vi "Keithley 2420 read resistance.vi"() -> ()   [LabVIEW 2014]
uses:
  Environmental Chamber LabVIEW and Instruments/Drivers and Software/LabVIEW 8.2 Drivers/keithley_24xx/Keithley 24XX/Public/Data/Read (Single Point).vi
  <vilib>/Utility/file.llb/Write To Spreadsheet File (string).vi
  Environmental Chamber LabVIEW and Instruments/Drivers and Software/keithley_24xx/Keithley 24XX/Keithley 24XX.lvlib
panel:
  in  "save?":bool
  in  "note":string
  in  "Stop Button":bool
  out "K-2420 2":cluster{"Resistance":sgl}(graph)
  in  "K2420 Applied Voltage (V)":dbl=0.1
  in  "K2420-range":dbl=1.0 format="%#_13g"
  in  "Enable Auto Range (T:Enable)":bool=TRUE
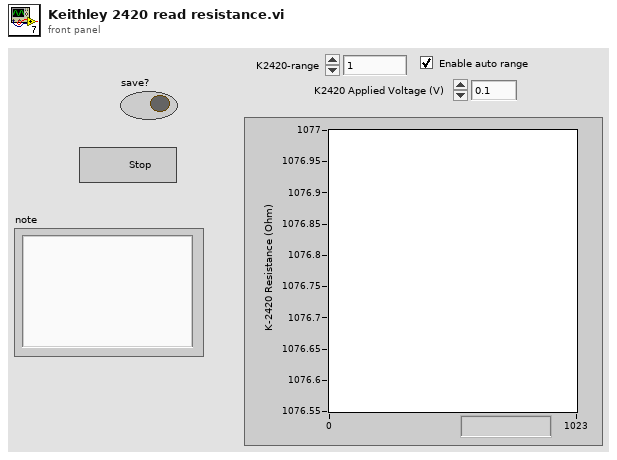
[diagram p1: front panel]
types:
  T1 = enum16{"open", "open or create", "create or replace", "create", "open (read only)"}
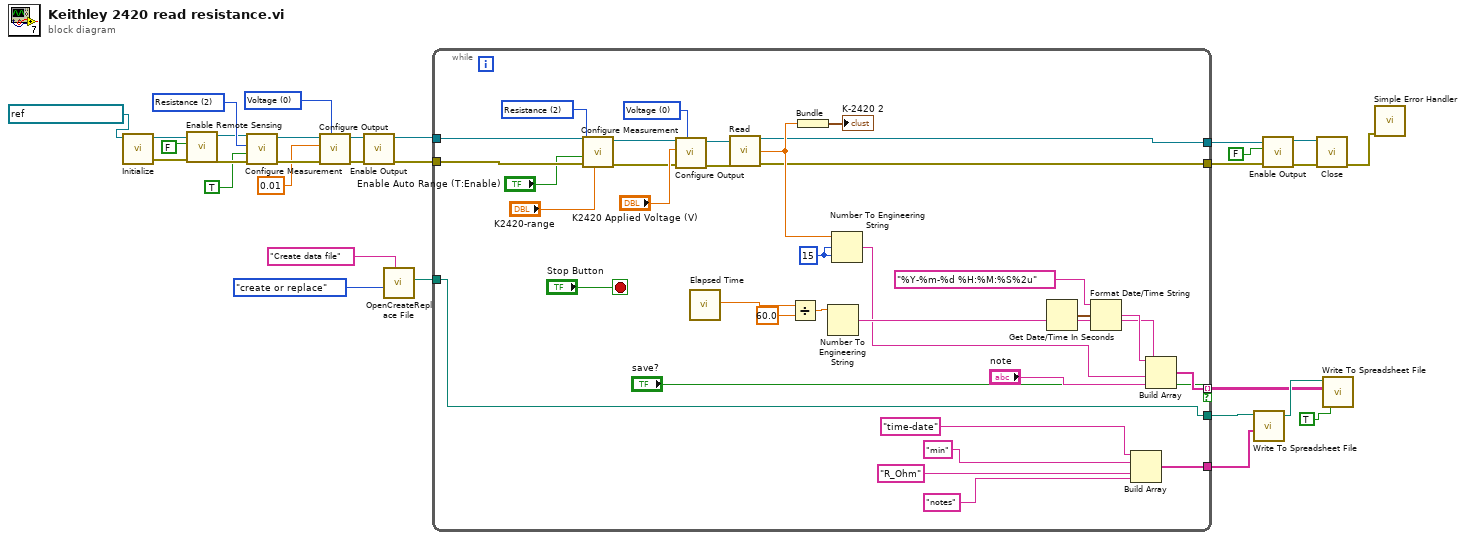
[diagram p0: block diagram]
diagram:
  w15 = u16 0 items=["Voltage", "Current"] ("Source Mode  (0: Voltage)")
  w20 = u16 2 items=["Volts", "Current", "Resistance"] ("Function (0: Volts)")
  n1 = call "Initialize.vi"("VISA resource name"=refnum<visa-resource-name> "GPIB1::24::INSTR") -> ("error out"=w11:errorcluster, "VISA resource name out"=w14:refnum<visa-resource-name>)  [unwired: 9 in]
  n2 = call "Enable Remote Sensing.vi"("error in (no error)"=w11, "Enable Remote Sensing (T: Enable)"=FALSE ("4-wire?"), "VISA resource name"=w14) -> ("error out"=w12:errorcluster, "VISA resource name out"=w13:refnum<visa-resource-name>)  [unwired: 7 in]
  n3 = call "Configure Measurement.vi"("error in (no error)"=w12, "Enable Auto Range (T:Enable)"=TRUE, "Function (0: Volts)"=w20, "VISA resource name"=w13) -> ("error out"=w19:errorcluster, "VISA resource name out"=w18:refnum<visa-resource-name>)  [unwired: 6 in]
  n4 = call "Configure Output.vi"("Source Mode  (0: Voltage)"=w15, "error in (no error)"=w19, "Output Level (0)"=0.01 ("K2420 Applied Voltage (V) 2"), "VISA resource name"=w18) -> ("error out"=w17:errorcluster, "VISA resource name out"=w16:refnum<visa-resource-name>)  [unwired: 6 in]
  n5 = call "Enable Output.vi"("error in (no error)"=w17, "VISA resource name"=w16) -> ("error out"=w29:errorcluster, "VISA resource name out"=w30:refnum<visa-resource-name>)  [unwired: 8 in]
  n6 = call "OpenCreateReplace File.vi"("prompt"="Create data file", "function (open:0)"=T1."create or replace") -> ("new file path"=w22:path)  [unwired: 6 in, 3 out]
  n7 = while {
    tunnel: [w62] -> w24 mode=indexing if="save?"
    tunnel: w30 -> [w58]
    tunnel: w29 -> [w57]
    tunnel: [w40] -> w25
    tunnel: w22 -> [w40]
    tunnel: [w44] -> w3
    tunnel: [w43] -> w2
    tunnel: [w36] -> w1
    stop <- "Stop Button" stop-if-true
    w45 = u16 2 items=["Volts", "Current", "Resistance"] ("Function (0: Volts)")
    w53 = u16 0 items=["Voltage", "Current"] ("Source Mode  (0: Voltage)")
    w54 = i16 15 ("width (-)")
    n8 = call "Configure Measurement.vi"("Manual Range (1.0)"="K2420-range", "error in (no error)"=w57, "Enable Auto Range (T:Enable)"="Enable Auto Range (T:Enable)", "Function (0: Volts)"=w45, "VISA resource name"=w58) -> ("error out"=w48:errorcluster, "VISA resource name out"=w49:refnum<visa-resource-name>)  [unwired: 5 in]
    n9 = call "Configure Output.vi"("Source Mode  (0: Voltage)"=w53, "error in (no error)"=w48, "Output Level (0)"="K2420 Applied Voltage (V)", "VISA resource name"=w49) -> ("error out"=w51:errorcluster, "VISA resource name out"=w52:refnum<visa-resource-name>)  [unwired: 6 in]
    n10 = call "Elapsed Time"() -> ("Elapsed Time (s)"=w42:dbl)  [unwired: 12 in, 7 out]
    n11 = call-poly "Read.vi"("VISA resource name"=w52, "error in (no error)"=w51) -> ("VISA resource name out"=w44:refnum<visa-resource-name>, "Resistance"=w55:sgl, "error out"=w43:errorcluster)  [unwired: 7 in, 4 out]
    n12 = Divide(x=w42, y=60.0) -> (x/y=w59:dbl)
    n13 = Bundle("Resistance"=w55) -> (→"K-2420 2":cluster{"Resistance":sgl})  [unwired: 1 in]
    n14 = Number To Engineering String ("elapsed time (min)")(4:w59) -> (0:w60:string)  [unwired: 3 in]
    n15 = Number To Engineering String(2:w54, 3:w54, 4:w55) -> (0:w38:string)  [unwired: 1 in]
    n16 = Get Date/Time In Seconds() -> (seconds since 1Jan1904=w64:timestamp)
    n17 = Format Date/Time String(time format string (%c)="%Y-%m-%d %H:%M:%S%2u", seconds (now)=w64) -> (date/time string=w61:string)  [unwired: 1 in]
    n18 = Build Array("time-date" ("note 2"), "min" ("note 2"), "R_Ohm" ("note 2"), "notes" ("note 2")) -> (w36:string[])
    n19 = Build Array(w61, w60, w38, "note") -> (w62:string[])
  }
  n20 = call-poly <vilib>:"Write To Spreadsheet File.vi"("1D data"=w1, "file path (dialog if empty)"=w25) -> ("new file path (Not A Path if cancelled)"=w28:path)  [unwired: 6 in]
  n21 = call "Enable Output.vi"("error in (no error)"=w2, "Enable Output (T: Enable)"=FALSE, "VISA resource name"=w3) -> ("error out"=w5:errorcluster, "VISA resource name out"=w7:refnum<visa-resource-name>)  [unwired: 7 in]
  n22 = call "Close.vi"("error in (no error)"=w5, "VISA resource name"=w7) -> ("error out"=w4:errorcluster)  [unwired: 9 in]
  n23 = call-poly <vilib>:"Write To Spreadsheet File.vi"("append to file? (new file:F)"=TRUE, "2D data"=w24, "file path (dialog if empty)"=w28) -> ()  [unwired: 5 in, 1 out]
  n24 = call <vilib>:"Simple Error Handler.vi"("error in (no error)"=w4) -> ()  [unwired: 4 in, 5 out]
